vi "Echo Canceling.vi"() -> ()   [LabVIEW 2023]
doc: "This example shows the application of using the complex cepstrum and inverse complex cepstrum to remove echoes in a signal.\n\nThe cepstrum of a signal that contains echoes has equally-spaced peaks at each echo delay. You can set the peaks in the cepstrum to zero and reconstruct the signal with echoes being removed. \n\nThis example simulates a signal with echoes and uses the TSA Complex Cepstrum VI and the TSA Inverse Complex Cepstrum VI to remove echoes from the signal.\n\n<b>Instructions:</b>\n1) Run this VI.\n2) Observe the reconstructed signal with echo removed."
uses:
  <vilib>/addons/Time Series Analysis/Utilities.llb/TSA Data.ctl
  <vilib>/Waveform/WDTOps.llb/WDT Number of Waveform Samples DBL.vi
  <vilib>/addons/Time Series Analysis/Correlation and Spectral Analysis.llb/TSA Complex Cepstrum (Waveform).vi
  <vilib>/addons/Time Series Analysis/Correlation and Spectral Analysis.llb/TSA Inverse Complex Cepstrum (Waveform).vi
  <vilib>/addons/_Advanced Signal Processing/NI_AdvSigProcTSA.lvlib
  <vilib>/measure/NI_MABase.lvlib
panel:
  in  "stop":bool
  out "Peak-Removed Cepstrum":cluster{"t0":dbl, "dt":dbl, "Cx":dbl[]}(graph)
  out "Reconstructed Signal":waveform(dbl)(graph)
  out "Complex Cepstrum":cluster{"t0":dbl, "dt":dbl, "C(t)":dbl[]}(graph)
  out "Signal with Echo":waveform(dbl)(graph)
  # "Overview: Shows the application of using the complex cepstrum and inverse complex cepstrum to remove echoes in a signal.\nRequirements: LabVIEW Full Development System, Advanced Signal Processing Toolkit\nInstructions: \n1. Run this VI.\n2. Observe the reconstructed signal with echo removed.\n3. Click Stop to stop the VI."
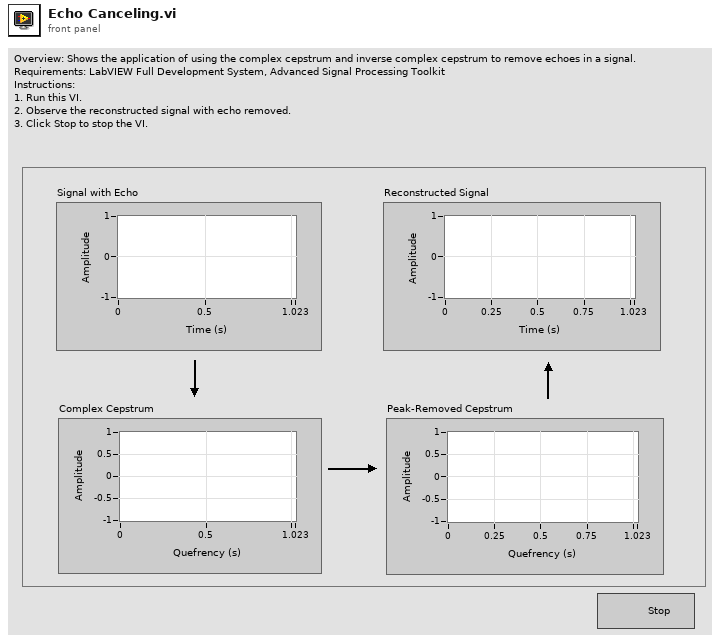
[diagram p1: front panel]
types:
  T1 = typedef "NI_AdvSigProcTSA.lvlib/TSA Data.ctl" = u16
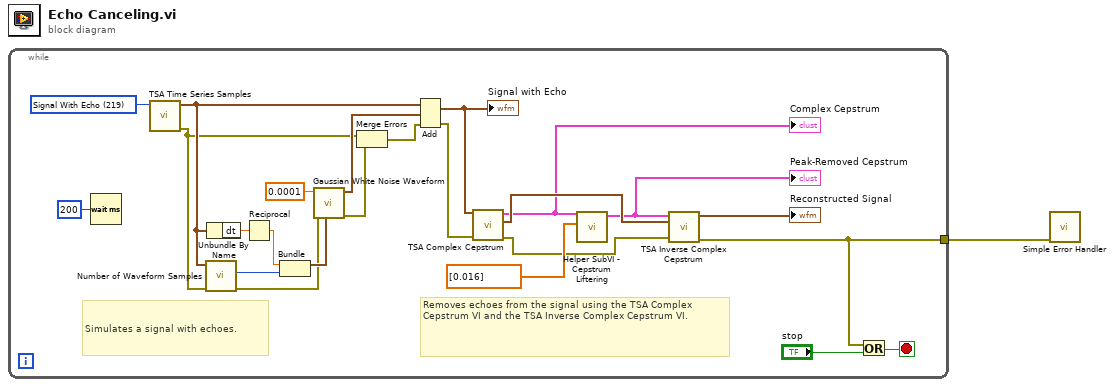
[diagram p0: block diagram]
diagram:
  n1 = while {
    tunnel: [w7] -> w1
    stop <- w18 stop-if-true
    w8 = T1 219 items=["Kobe Earthquake"=201, "EEG"=210, "Bearing Vibration (simulated)"=211, "Period Product Sales"=214, "Beam Vibration (nonlinear)"=217, "Beam Vibration (linear)"=218, "Signal With Echo"=219, "Engine Knocking"=220, "Power Line"=221, "-"=200, "Beam Deflections (multivariate)"=207, "Structure Vibration (multivariate)"=208, "Human MEG (multivariate)"=222] ("data")
    # "Removes echoes from the signal using the TSA Complex Cepstrum VI and the TSA Inverse Complex Cepstrum VI."
    # "Simulates a signal with echoes."
    n2 = Wait (ms)(milliseconds to wait=u32 200 ("millisecond multiple")) -> ()  [unwired: 1 out]
    n3 = call <vilib>:"TSA Time Series Samples.vi"("data"=w8) -> ("error out"=w4:errorcluster, "univariate time series"=w10:waveform(dbl))  [unwired: 1 in, 8 out]
    n4 = call-poly <vilib>:"Number of Waveform Samples.vi"("error in (no error)"=w4, "waveform in"=w10) -> ("error out"=w5:errorcluster, "number of samples"=w13:i32)  [unwired: 8 out]
    n5 = Unbundle By Name(w10) -> ("dt"=w14:dbl)
    n6 = Reciprocal(x=w14) -> (1/x=w9:dbl)
    n7 = Bundle(w9, "number of samples"=w13) -> (w12:cluster{dbl, "number of samples":i32})  [unwired: 1 out]
    n8 = call <vilib>:"Gaussian White Noise Waveform.vi"("sampling info"=w12, "error in (no error)"=w5, "standard deviation"=0.0001) -> ("error out"=w3:errorcluster, "signal out"=w15:waveform(dbl))  [unwired: 2 in, 5 out]
    n9 = Merge Errors(w4, w3) -> (w2:errorcluster)
    n10 = Add(1:w15, 2:w10, 4:w2) -> (0:w16:waveform(dbl), 3:w6:errorcluster)
    "Signal with Echo" <- w16
    n11 = call-poly <vilib>:"TSA Complex Cepstrum.vi"("error in (no error)"=w6, "Xt"=w16) -> ("error out"=w20:errorcluster, "phase info"=w25:cluster{"DC":dbl, "Nyquist":dbl}, "cepstrum"=w24:cluster{"t0":dbl, "dt":dbl, "C(t)":dbl[]})  [unwired: 7 out]
    "Complex Cepstrum" <- w24
    n12 = call "Helper SubVI - Cepstrum Liftering.vi"("base t"=dbl[] [0.016], "cepstrum in"=w24) -> ("cepstrum out"=w23:cluster{"t0":dbl, "dt":dbl, "Cx":dbl[]})  [unwired: 7 in, 2 out]
    "Peak-Removed Cepstrum" <- w23
    n13 = call-poly <vilib>:"TSA Inverse Complex Cepstrum.vi"("error in (no error)"=w20, "phase info"=w25, "cepstrum"=w23) -> ("error out"=w7:errorcluster, "Xt"=→"Reconstructed Signal":waveform(dbl))  [unwired: 7 out]
    n14 = Or(x=w7, y="stop") -> (x .or. y?=w18:bool)
  }
  n15 = call <vilib>:"Simple Error Handler.vi"("error in (no error)"=w1) -> ()  [unwired: 1 in, 8 out]
